vi "Target Focus POLARIS Vision.vi"() -> ()   [LabVIEW 2009]
uses:
  XDisplay/POLARIS IMAQ Display.xctl
  Analyze Classes/Width Method.ctl
  Analyze Classes/Analyze Fluence/Analyze Fluence.lvclass
  Analyze Classes/Analyze Q-Factor/Analyze q-Factor.lvclass
  XDisplay/Properties/ImageSource.ctl
  IMAQdx Cam/IMAQdx Cam.lvclass
  Utility/POLARIS Vision utility.lvlib
panel:
  in  "User Prefix":string
  out "error load data":errorcluster
  in  "Camera Name":string
  in  "Amplifier":u16(ring) items=["CW", "A2", "A2 1.6x", "A3", "A4", "A5"]
  in  "Compressor eff.":dbl=0.63
  in  "stop2":bool
  out "I [W/cm^2]":dbl format="%#.2g"
  in  "Pulse duration [fs]":dbl=150.0
  in  "SW Trigger":bool
  out "error out":errorcluster
  out "q-Factor":dbl format="%#_3g"
  out "Focus/µm^2":dbl format="%#.1g"
  in  "Method":T1
  in  "Size of hotest Region":i32=10
  in  "Energy  A4 or A5 [J]":dbl=10.0
  out "error save settings":errorcluster
  in  "Config Dir":path
  in  "Results String":string
  in  "WorkDir":path
  out "XDisplay":cluster{"Image":T2}(xcontrol)
  in  "stop":bool
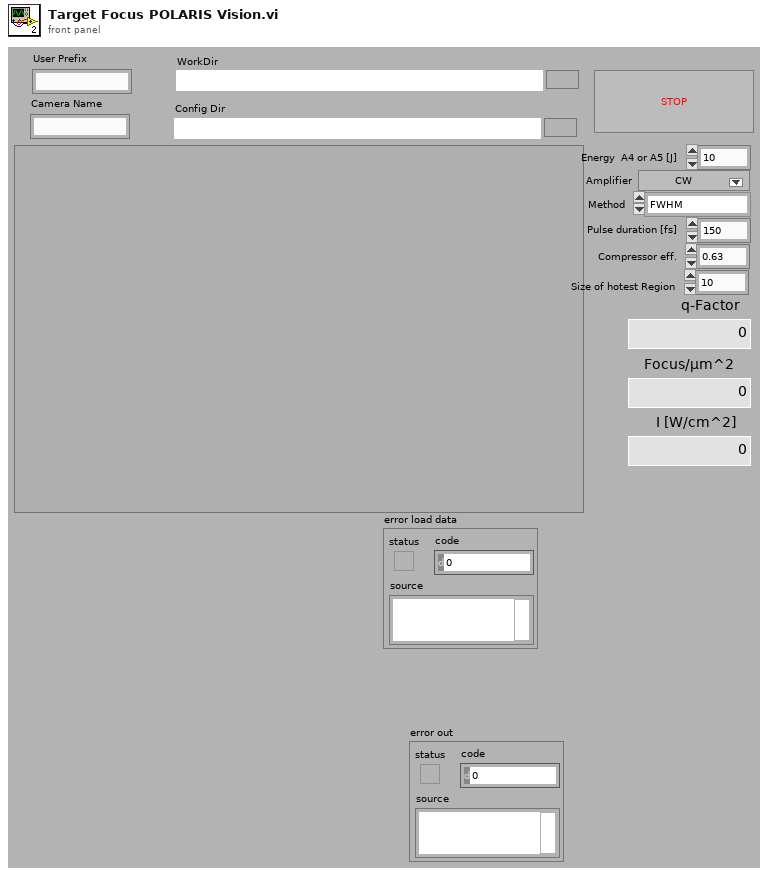
[diagram p1: front panel]
types:
  T1 = typedef "Width Method.ctl" = enum16{"FWHM", "1/e", "1/e^2", "80%", "90%"}
  T2 = typedef "IMAQ Image.ctl" = refnum<image>
  T3 = typedef "POLARIS IMAQ Display.xctl/ImageSource.ctl" = enum16{"Camera", "File"}
  T4 = typedef "Image Type" = u32
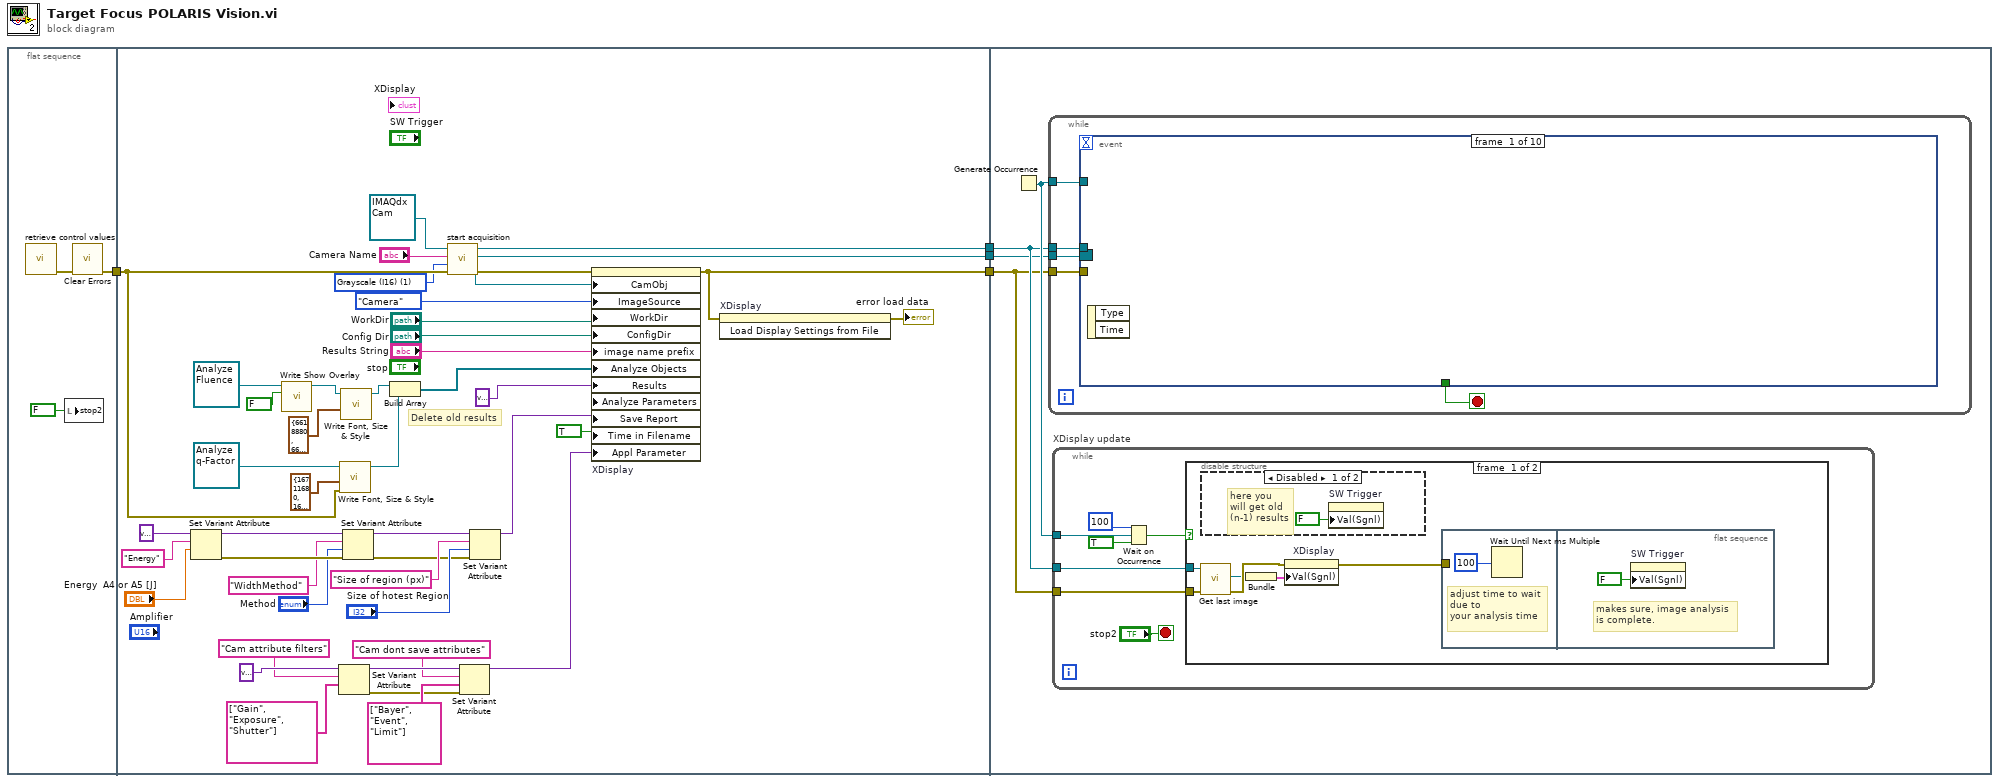
[diagram p0: block diagram]
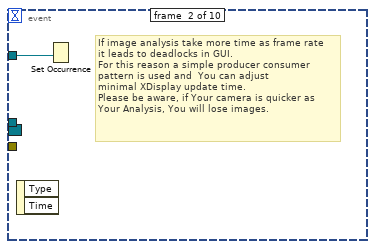
[diagram p4: hidden frame]
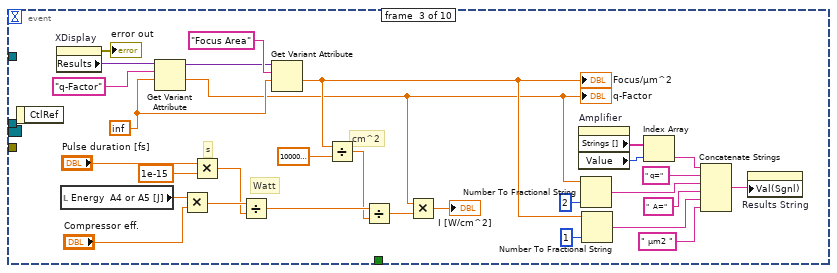
[diagram p5: hidden frame]
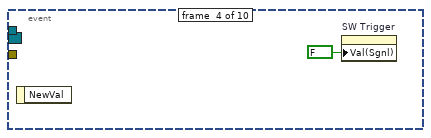
[diagram p6: hidden frame]
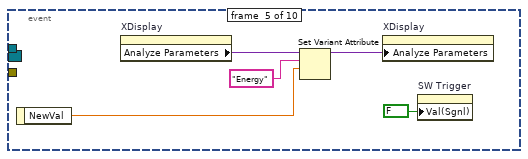
[diagram p7: hidden frame]
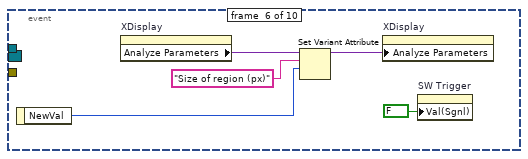
[diagram p8: hidden frame]
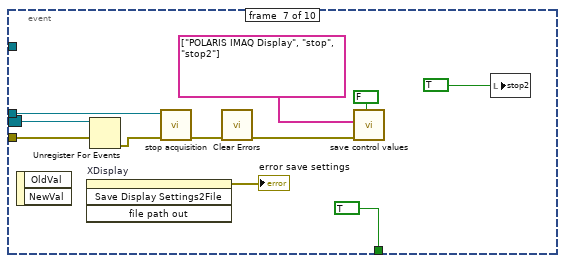
[diagram p9: hidden frame]
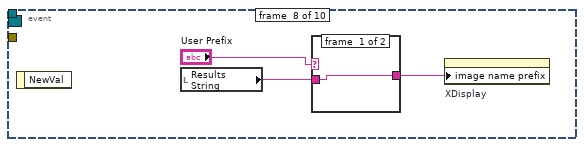
[diagram p10: hidden frame]
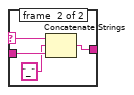
[diagram p11: hidden frame]
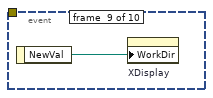
[diagram p12: hidden frame]
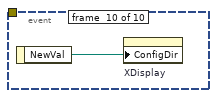
[diagram p13: hidden frame]
diagram:
  n1 = flat-sequence {
    tunnel: [w6] -> w4
    tunnel: w4 -> [w40]
    tunnel: [w25] -> w3
    tunnel: [w24] -> w2
    tunnel: [w23] -> w1
    tunnel: w3 -> [w54]
    tunnel: w2 -> [w53]
    tunnel: w1 -> [w52]
    frame #0 {
      n2 = call "retrieve control values.vi"() -> ("error out"=w7:errorcluster)  [unwired: 10 in, 1 out]
      n3 = local write "stop2"(FALSE ("stop2")) -> ()
      n4 = call <vilib>:"Clear Errors.vi"("error in (no error)"=w7) -> ("error out"=w6:errorcluster)  [unwired: 6 in]
    }
    frame #1 {
      w28 = TRUE ("Time in Filename")
      w8 = T4 1 items=["Grayscale (U8)", "Grayscale (I16)", "Grayscale (SGL)", "Complex (CSG)", "RGB (U32)", "HSL (U32)", "RGB (U64)", "Grayscale (U16)"] ("Image Type")
      # "Delete old results"
      n5 = Set Variant Attribute(Variant=variant ("variant"), name="Energy", value="Energy  A4 or A5 [J]") -> (Variant out=w37:variant, error out=w39:errorcluster)  [unwired: 1 in, 1 out]
      n6 = call-dynamic "Write Show Overlay.vi"("Overlay?"=FALSE, "Analyze BaseClass in"=refnum<class "Analyze Fluence.lvclass"> refnum ("Analyze Fluence.lvclass")) -> ("Analyze BaseClass out"=w19:refnum<class "Analyze Fluence.lvclass">)  [unwired: 8 in, 1 out]
      n7 = Set Variant Attribute(Variant=variant ("Results"), name="Cam attribute filters", value=string[] ["Gain", "Exposure", "Shutter"] ("Filters")) -> (Variant out=w12:variant, error out=w10:errorcluster)  [unwired: 1 in, 1 out]
      n8 = call-dynamic "Write Font, Size & Style.vi"("error in (no error)"=w40, "Overlay colors"=cluster{"Border":u32, "Text":u32} {"Border"=16711680, "Text"=16448250}, "Analyze BaseClass in"=refnum<class "Analyze q-Factor.lvclass"> refnum ("Analyze Q-Factor.lvclass")) -> ("Analyze BaseClass out"=w43:refnum<class "Analyze q-Factor.lvclass">)  [unwired: 7 in, 1 out]
      n9 = call-dynamic "Write Font, Size & Style.vi"("Overlay colors"=cluster{"Border":u32, "Text":u32} {"Border"=6618880, "Text"=6618880}, "Analyze BaseClass in"=w19) -> ("Analyze BaseClass out"=w18:refnum<class "Analyze Fluence.lvclass">)  [unwired: 8 in, 1 out]
      n10 = Set Variant Attribute(Variant=w37, name="WidthMethod", value="Method", error in=w39) -> (Variant out=w32:variant, error out=w17:errorcluster)  [unwired: 1 out]
      n11 = Build Array(w18, w43) -> (w42:refnum<class "Analyze BaseClass.lvclass">[])
      n12 = call-dynamic "start acquisition.vi"("error in (no error)"=w40, "Image Type"=w8, "Camera Name"="Camera Name", "IMAQdx Cam in"=refnum<class "IMAQdx Cam.lvclass"> refnum ("IMAQdx Cam.lvclass")) -> ("error out"=w48:errorcluster, "Event Registration Refnum"=w24:refnum<event-registration>, "IMAQdx Cam out"=w25:refnum<class "IMAQdx Cam.lvclass">)  [unwired: 5 in]
      n13 = Set Variant Attribute(Variant=w12, name="Cam dont save attributes", value=string[] ["Bayer", "Event", "Limit"] ("do not save"), error in=w10) -> (Variant out=w9:variant)  [unwired: 2 out]
      n14 = Set Variant Attribute(Variant=w32, name="Size of region (px)", value="Size of hotest Region", error in=w17) -> (Variant out=w31:variant)  [unwired: 2 out]
      n15 = property on="XDisplay" class="POLARIS IMAQ Display (strict)"(error in=w48, "CamObj"=w25, "ImageSource"=ImageSource."Camera", "WorkDir"="WorkDir", "ConfigDir"="Config Dir", "image name prefix"="Results String", "Analyze Objects"=w42, "Results"=variant, "Analyze Parameters"=w31, "Save Report"=w28, "Time in Filename"=w28, "Appl Parameter"=w9) -> (error out=w23:errorcluster)  [unwired: 1 in, 1 out]
      n16 = invoke on="XDisplay" class="POLARIS IMAQ Display (strict)" method="Load Display Settings from File"(error in=w23) -> (error out=→"error load data":errorcluster)  [unwired: 2 in, 2 out]
    }
    frame #2 {
      n17 = Generate Occurrence() -> (w55:refnum<k4>)
      n18 = while {
        tunnel: w54 -> [w75]
        tunnel: w53 -> [w74]
        tunnel: w52 -> [w73]
        tunnel: w55 -> [w72]
        stop <- w76 stop-if-true
        n19 = event shown="[2] \"SW Trigger\": Value Change" {
          selector: w74 -> [_ _ _ _ _ _ w126 _ _ _]
          dyn-events: _ -> [_ _ _ _ _ _ _ _ _ _]
          timeout: _ -> [_ _ _ _ _ _ _ _ _ _]
          tunnel: [_ _ _ _ _ _ TRUE _ _ _] -> w76
          tunnel: w75 -> [_ _ _ _ _ _ w127 _ _ _]
          tunnel: w73 -> [_ _ _ _ _ _ w125 _ _ _]
          tunnel: w72 -> [_ w77 _ _ _ _ _ _ _ _]
          event #0 {
            n20 = event-data() -> ()  [unwired: 1 in, 2 out]
          }
          event #1 {
            # "If image analysis take more time as frame rate\nit leads to deadlocks in GUI.\nFor this reason a simple producer consumer \npattern is used and  You can adjust \nminimal XDisplay update time.\nPlease be aware, if Your camera is quicker as\nYour Analysis, You will lose images."
            n21 = event-data() -> ()  [unwired: 1 in, 2 out]
            n22 = Set Occurrence(w77) -> ()
          }
          event #2 {
            w103 = inf
            # "cm^2"
            # "s"
            # "Watt"
            n23 = event-data() -> ()  [unwired: 1 in, 1 out]
            n24 = property on="XDisplay" class="POLARIS IMAQ Display (strict)"() -> (error out=→"error out":errorcluster, "Results"=w106:variant)  [unwired: 2 in, 1 out]
            n25 = local read "Energy  A4 or A5 [J]"() -> (w101:dbl)
            n26 = Get Variant Attribute(Variant=w106, name="q-Factor", default value (empty Variant)=w103) -> (duplicate Variant=w104:variant, value=w78:dbl)  [unwired: 1 in, 2 out]
            "q-Factor" <- w78
            n27 = Multiply(x=w101, y="Compressor eff.") -> (x*y=w99:dbl)
            n28 = Multiply(x="Pulse duration [fs]", y=1e-15) -> (x*y=w97:dbl)
            n29 = Divide(x=w99, y=w97) -> (x/y=w95:dbl)
            n30 = Get Variant Attribute(Variant=w104, name="Focus Area", default value (empty Variant)=w103) -> (value=w82:dbl)  [unwired: 1 in, 3 out]
            "Focus/µm^2" <- w82
            n31 = Divide(x=w82, y=100000000.0) -> (x/y=w93:dbl)
            n32 = Divide(x=w95, y=w93) -> (x/y=w92:dbl)
            n33 = Multiply(x=w78, y=w92) -> (x*y=→"I [W/cm^2]":dbl)
            n34 = property on="Amplifier" class="Ring (strict)"() -> ("Strings []"=w90:string[], "Value"=w91:u16)  [unwired: 2 in, 2 out]
            n35 = Number To Fractional String(number=w78, precision (6)=i16 2 ("Genauigkeit (6)")) -> (F-format string=w87:string)  [unwired: 2 in]
            n36 = Number To Fractional String(number=w82, precision (6)=i16 1 ("Genauigkeit (6)")) -> (F-format string=w81:string)  [unwired: 2 in]
            n37 = Index Array(array=w90, index=w91) -> (element=w89:string)
            n38 = Concatenate Strings(w89, " q=" ("String"), w87, "  A=" ("String"), w81, " µm2 " ("String")) -> (w79:string)
            n39 = property on="Results String" class="Str"("Val(Sgnl)"=w79) -> ()  [unwired: 2 in, 2 out]
          }
          event #3 {
            n40 = event-data() -> ()  [unwired: 1 in, 1 out]
            n41 = property on="SW Trigger" class="Bool (strict)"("Val(Sgnl)"=FALSE ("Value (Signaling)")) -> ()  [unwired: 2 in, 2 out]
          }
          event #4 {
            n42 = event-data() -> ("NewVal"=w110:dbl)  [unwired: 1 in]
            n43 = property on="XDisplay" class="POLARIS IMAQ Display (strict)"() -> ("Analyze Parameters"=w113:variant)  [unwired: 2 in, 2 out]
            n44 = Set Variant Attribute(Variant=w113, name="Energy", value=w110) -> (Variant out=w111:variant)  [unwired: 1 in, 2 out]
            n45 = property on="XDisplay" class="POLARIS IMAQ Display (strict)"("Analyze Parameters"=w111) -> ()  [unwired: 2 in, 2 out]
            n46 = property on="SW Trigger" class="Bool (strict)"("Val(Sgnl)"=FALSE ("Value (Signaling)")) -> ()  [unwired: 2 in, 2 out]
          }
          event #5 {
            n47 = event-data() -> ("NewVal"=w115:i32)  [unwired: 1 in]
            n48 = property on="XDisplay" class="POLARIS IMAQ Display (strict)"() -> ("Analyze Parameters"=w118:variant)  [unwired: 2 in, 2 out]
            n49 = Set Variant Attribute(Variant=w118, name="Size of region (px)", value=w115) -> (Variant out=w116:variant)  [unwired: 1 in, 2 out]
            n50 = property on="XDisplay" class="POLARIS IMAQ Display (strict)"("Analyze Parameters"=w116) -> ()  [unwired: 2 in, 2 out]
            n51 = property on="SW Trigger" class="Bool (strict)"("Val(Sgnl)"=FALSE ("Value (Signaling)")) -> ()  [unwired: 2 in, 2 out]
          }
          event #6 {
            n52 = event-data() -> ()  [unwired: 1 in, 2 out]
            n53 = invoke on="XDisplay" class="POLARIS IMAQ Display (strict)" method="Save Display Settings2File"() -> (error out=→"error save settings":errorcluster)  [unwired: 4 in, 3 out]
            n54 = Unregister For Events(event registration refnum=w126, error in=w125) -> (error out=w128:errorcluster)
            n55 = call-dynamic "stop acquisition.vi"("error in (no error)"=w128, "IMAQdx Cam in"=w127) -> ("error out"=w124:errorcluster)  [unwired: 8 in, 1 out]
            n56 = call <vilib>:"Clear Errors.vi"("error in (no error)"=w124) -> ("error out"=w123:errorcluster)  [unwired: 6 in]
            n57 = call "save control values.vi"("Append timestamp (true)"=FALSE, "error in"=w123, "Dont save"=string[] ["POLARIS IMAQ Display", "stop", "stop2"]) -> ()  [unwired: 5 in, 2 out]
            n58 = local write "stop2"(TRUE ("stop2")) -> ()
          }
          event #7 {
            n59 = event-data() -> ()  [unwired: 1 in, 1 out]
            n60 = local read "Results String"() -> (w130:string)
            n61 = case shown="\"True\", Default" "User Prefix" {
              selector: "User Prefix" -> [_ w134]
              tunnel: w130 -> [w133 w137]
              tunnel: [w133 w136] -> w132
              frame #0 {
              }
              frame #1 {
                n62 = Concatenate Strings(w134, "_" ("string"), w137) -> (w136:string)
              }
            }
            n63 = property on="XDisplay" class="POLARIS IMAQ Display (strict)"("image name prefix"=w132) -> ()  [unwired: 2 in, 2 out]
          }
          event #8 {
            n64 = event-data() -> ("NewVal"=w138:path)  [unwired: 1 in]
            n65 = property on="XDisplay" class="POLARIS IMAQ Display (strict)"("WorkDir"=w138) -> ()  [unwired: 2 in, 2 out]
          }
          event #9 {
            n66 = event-data() -> ("NewVal"=w139:path)  [unwired: 1 in]
            n67 = property on="XDisplay" class="POLARIS IMAQ Display (strict)"("ConfigDir"=w139) -> ()  [unwired: 2 in, 2 out]
          }
        }
      }
      n68 = while "XDisplay update" {
        tunnel: w55 -> [w62]
        tunnel: w54 -> [w59]
        tunnel: w52 -> [w58]
        stop <- "stop2" stop-if-true
        n69 = Wait on Occurrence(1:TRUE ("ignore previous (T)"), 2:w62, 3:100 ("ms timeout (-1)")) -> (0:w60:bool)
        n70 = case shown="False" w60 {
          tunnel: w59 -> [w65 _]
          tunnel: w58 -> [w64 _]
          frame #0 {
            n71 = call-dynamic "Get last image.vi"("error in (no error)"=w64, "IMAQdx Cam in"=w65) -> ("error out"=w67:errorcluster, "Image Out"=w66:T2)  [unwired: 7 in, 1 out]
            n72 = disable-structure shown="Disabled" {
              frame #0 {
                # "here you\nwill get old \n(n-1) results"
                n73 = property on="SW Trigger" class="Bool (strict)"("Val(Sgnl)"=FALSE ("Value (Signaling)")) -> ()  [unwired: 2 in, 2 out]
              }
              frame #1 {
              }
            }
            n74 = Bundle("Image Out"=w66) -> (w68:cluster{"Image Out":T2})  [unwired: 1 in]
            n75 = property on="XDisplay" class="POLARIS IMAQ Display (strict)"(error in=w67, "Val(Sgnl)"=w68) -> (error out=w63:errorcluster)  [unwired: 1 in, 1 out]
            n76 = flat-sequence {
              tunnel: w63 -> [_]
              frame #0 {
                # "adjust time to wait\ndue to \nyour analysis time"
                n77 = Wait Until Next ms Multiple(millisecond multiple=u32 100 ("milliseconds to wait")) -> ()  [unwired: 1 out]
              }
              frame #1 {
                # "makes sure, image analysis\nis complete."
                n78 = property on="SW Trigger" class="Bool (strict)"("Val(Sgnl)"=FALSE ("Value (Signaling)")) -> ()  [unwired: 2 in, 2 out]
              }
            }
          }
          frame #1 {
          }
        }
      }
    }
  }
